vi "terminate.vi"(8 "error in (no error)":errorcluster, 11 "GenericPlugin in":refnum<class "FPGAWrapperMM140723Galvo.lvclass">) -> (0 "error out":errorcluster, 3 "GenericPlugin out":refnum<class "FPGAWrapperMM140723Galvo.lvclass">)   [LabVIEW 2010, in "FPGAWrapperMM140723Galvo.lvclass"]
doc: "The dynamic dispatch version of this VI terminates the plug-in object by releasing all of its resources."
uses:
  FPGAWrapperMM140723Galvo.lvclass
  GenericFPGAWrapper/GenericFPGAWrapper/GenericFPGAWrapper.lvclass
  type definitions/command_enum.ctl
  class_data.vi
  common/classes/ErrorController/ErrorController/class_data.vi
  common/classes/ErrorController/ErrorController/ErrorController.lvclass
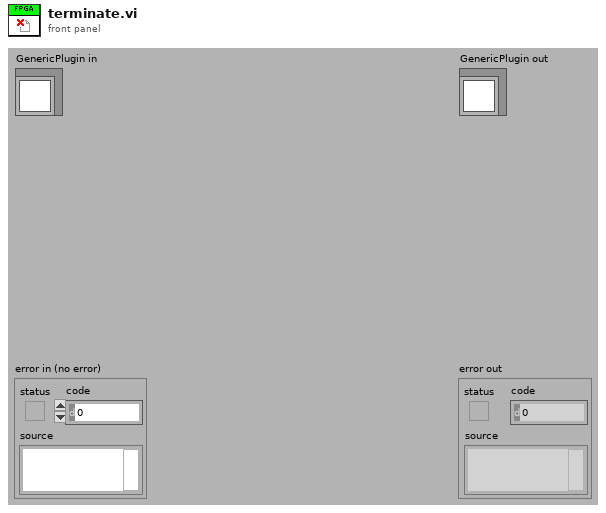
[diagram p1: front panel]
types:
  T1 = typedef "command_enum.ctl" = enum16{"NULL", "update", "start", "stop", "reset", "shut-down"}
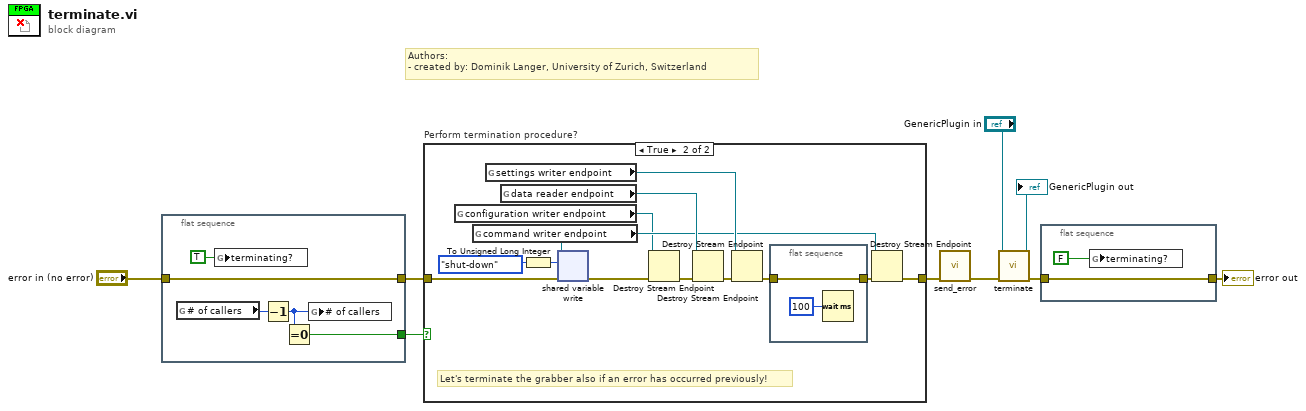
[diagram p0: block diagram]
diagram:
  # "Authors: \n- created by: Dominik Langer, University of Zurich, Switzerland"
  n1 = flat-sequence {
    tunnel: [w14] -> w3
    tunnel: [w13] -> w2
    tunnel: "error in (no error)" -> [w14]
    frame #0 {
      n2 = global read "class_data.vi" "# of callers"() -> (w12:i32)
      n3 = global write "class_data.vi" "terminating?"(TRUE ("terminating?")) -> ()
      n4 = Decrement(x=w12) -> (x-1=w11:i32)
      n5 = Equal To 0?(x=w11) -> (x = 0?=w13:bool)
      n6 = global write "class_data.vi" "# of callers"(w11) -> ()
    }
  }
  n7 = case "Perform termination procedure?" shown="True" w2 {
    tunnel: w3 -> [w15 w26]
    tunnel: [w15 w23] -> w1
    frame False {
    }
    frame True {
      # "Let's terminate the grabber also if an error has occurred previously!"
      n8 = global read "class_data.vi" "configuration writer endpoint"() -> (w18:refnum<k21>)
      n9 = global read "class_data.vi" "command writer endpoint"() -> (w21:refnum<k21>)
      n10 = global read "class_data.vi" "settings writer endpoint"() -> (w22:refnum<k21>)
      n11 = global read "class_data.vi" "data reader endpoint"() -> (w25:refnum<k21>)
      n12 = To Unsigned Long Integer(number=command_enum."shut-down" ("command")) -> (unsigned 32bit integer=w28:u32)
      n13 = shared-variable-write(w21, w26, w28) -> (w17:errorcluster)  [unwired: 1 in, 2 out]
      n14 = Destroy Stream Endpoint(8:w17, 11:w18) -> (0:w16:errorcluster)
      n15 = Destroy Stream Endpoint(8:w16, 11:w25) -> (0:w24:errorcluster)
      n16 = Destroy Stream Endpoint(8:w24, 11:w22) -> (0:w20:errorcluster)
      n17 = flat-sequence {
        tunnel: [w30] -> w19
        tunnel: w20 -> [w30]
        frame #0 {
          n18 = Wait (ms)(milliseconds to wait=u32 100) -> ()  [unwired: 1 out]
        }
      }
      n19 = Destroy Stream Endpoint(8:w19, 11:w21) -> (0:w23:errorcluster)
    }
  }
  n20 = call "send_error.vi"("error in (no error)"=w1) -> ("error out"=w6:errorcluster)  [unwired: 10 in]
  n21 = call-parent "terminate.vi"("error in (no error)"=w6, "GenericPlugin in"="GenericPlugin in") -> ("error out"=w5:errorcluster, "GenericPlugin out"=→"GenericPlugin out":refnum<class "FPGAWrapperMM140723Galvo.lvclass">)  [unwired: 8 in]
  n22 = flat-sequence {
    tunnel: [w32] -> w4
    tunnel: w5 -> [w32]
    frame #0 {
      n23 = global write "class_data.vi" "terminating?"(FALSE ("ready for initialise?")) -> ()
    }
  }
  "error out" <- w4
